vi "RunFullWormRails.vi"() -> ()   [LabVIEW 2019]
uses:
  Parameters.ctl
  FullWormRails/FullWormRailsInputCluster.ctl
  FullWormRails.lvclass
  D:/Github_repos/ProjectAPI/LabviewVIs/StimulusObject.lvclass
panel:
  in  "FullWormRailsInputCluster":T1={"Constant Intensity (uW/mm^2, negative is blue)"=0.0, "dot radius (mm)"=0.3, "Intensities (uW/mm^2, negative is blue)"=[], "Durations (s)"=[], "Inter trigger interval (s)"=10.0}
  out "error IO":errorcluster
  in  "SSH password 2":string
  in  "SSH user name 2":string
  in  "Start":bool
  in  "Wait Before Recording (s)":u32
  in  "SSH password":string
  in  "username@della.princeton.edu":string
  in  "Last Experiment of the Day":bool
  in  "Tags":string
  out "Parameters":T2 {"FW_WormLengthSD" format="%#.6e"}
  # "Faux Worm Drawing"
  # "Tracking"
  # "Temporal Calibration"
  # "Stimulus Generation"
  # "Median Filtering"
  # "Experimental Settings"
  # "Camera and Projector Settings"
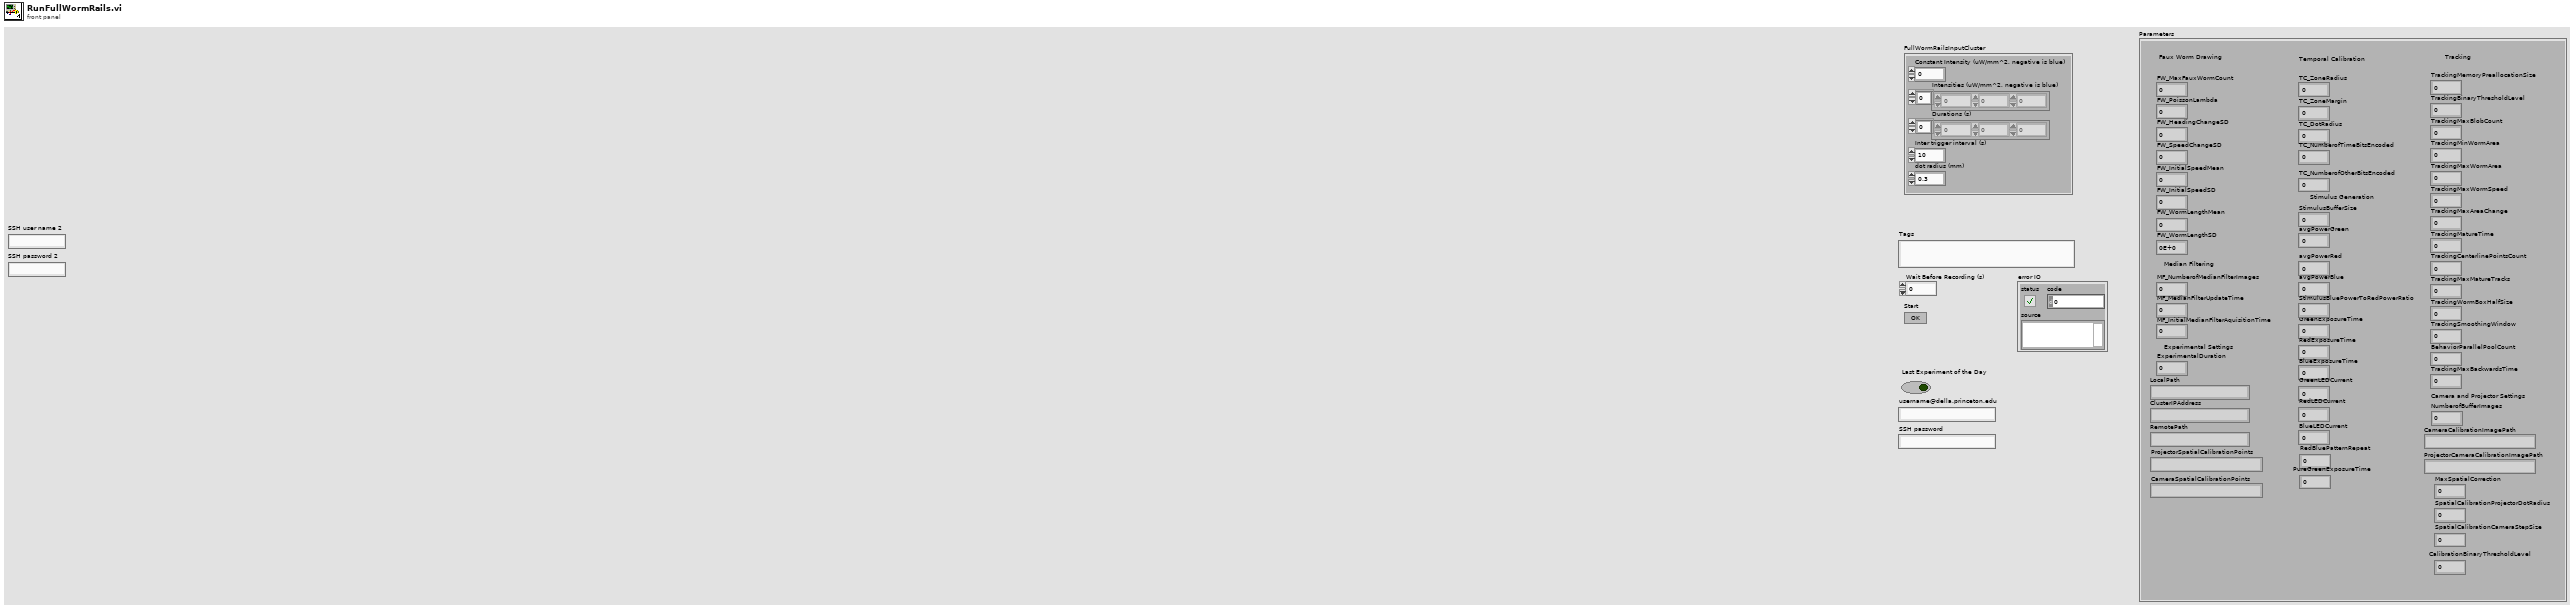
[diagram p1: front panel]
types:
  T1 = typedef "FullWormRails.lvclass/FullWormRailsInputCluster.ctl" = cluster{"Constant Intensity (uW/mm^2, negative is blue)":sgl, "dot radius (mm)":sgl, "Intensities (uW/mm^2, negative is blue)":sgl[], "Durations (s)":sgl[], "Inter trigger interval (s)":dbl}
  T2 = typedef "Parameters.ctl" = cluster{"FW_MaxFauxWormCount":i32, "FW_PoissonLambda":dbl, "FW_HeadingChangeSD":dbl, "FW_SpeedChangeSD":dbl, "FW_InitialSpeedMean":dbl, "FW_InitialSpeedSD":dbl, "FW_WormLengthMean":dbl, "FW_WormLengthSD":dbl, "MF_NumberofMedianFilterImages":i32, "MF_MedianFilterUpdateTime":i32, "MF_InitialMedianFilterAquisitionTime":dbl, "ExperimentalDuration":i32, "TC_ZoneRadius":i32, "TC_ZoneMargin":i32, "TC_DotRadius":dbl, "TC_NumberofTimeBitsEncoded":i32, "TC_NumberofOtherBitsEncoded":i32, "NumberofBufferImages":sgl, "CameraCalibrationImagePath":string, "ProjectorCameraCalibrationImagePath":string, "StimulusBufferSize":i32, "TrackingMemoryPreallocationSize":i32, "TrackingBinaryThresholdLevel":sgl, "TrackingMaxBlobCount":i32, "TrackingMinWormArea":dbl, "TrackingMaxWormArea":dbl, "TrackingMaxWormSpeed":dbl, "TrackingMaxAreaChange":dbl, "TrackingMatureTime":i32, "TrackingCenterlinePointsCount":i32, "TrackingMaxMatureTracks":i32, "TrackingWormBoxHalfSize":i32, "TrackingSmoothingWindow":i32, "BehaviorParallelPoolCount":i32, "LocalPath":string, "GreenExposureTime":i32, "RedExposureTime":i32, "BlueExposureTime":i32, "ClusterIPAddress":string, "RemotePath":string, "GreenLEDCurrent":u8, "RedLEDCurrent":u8, "BlueLEDCurrent":u8, "avgPowerGreen":sgl, "avgPowerRed":sgl, "avgPowerBlue":sgl, "StimulusBluePowerToRedPowerRatio":sgl, "TrackingMaxBackwardsTime":i32, "MaxSpatialCorrection":dbl, "ProjectorSpatialCalibrationPoints":string, "SpatialCalibrationProjectorDotRadius":i32, "SpatialCalibrationCameraStepSize":dbl, "CameraSpatialCalibrationPoints":string, "CalibrationBinaryThresholdLevel":dbl, "RedBluePatternRepeat":i32, "PureGreenExposureTime":i32}
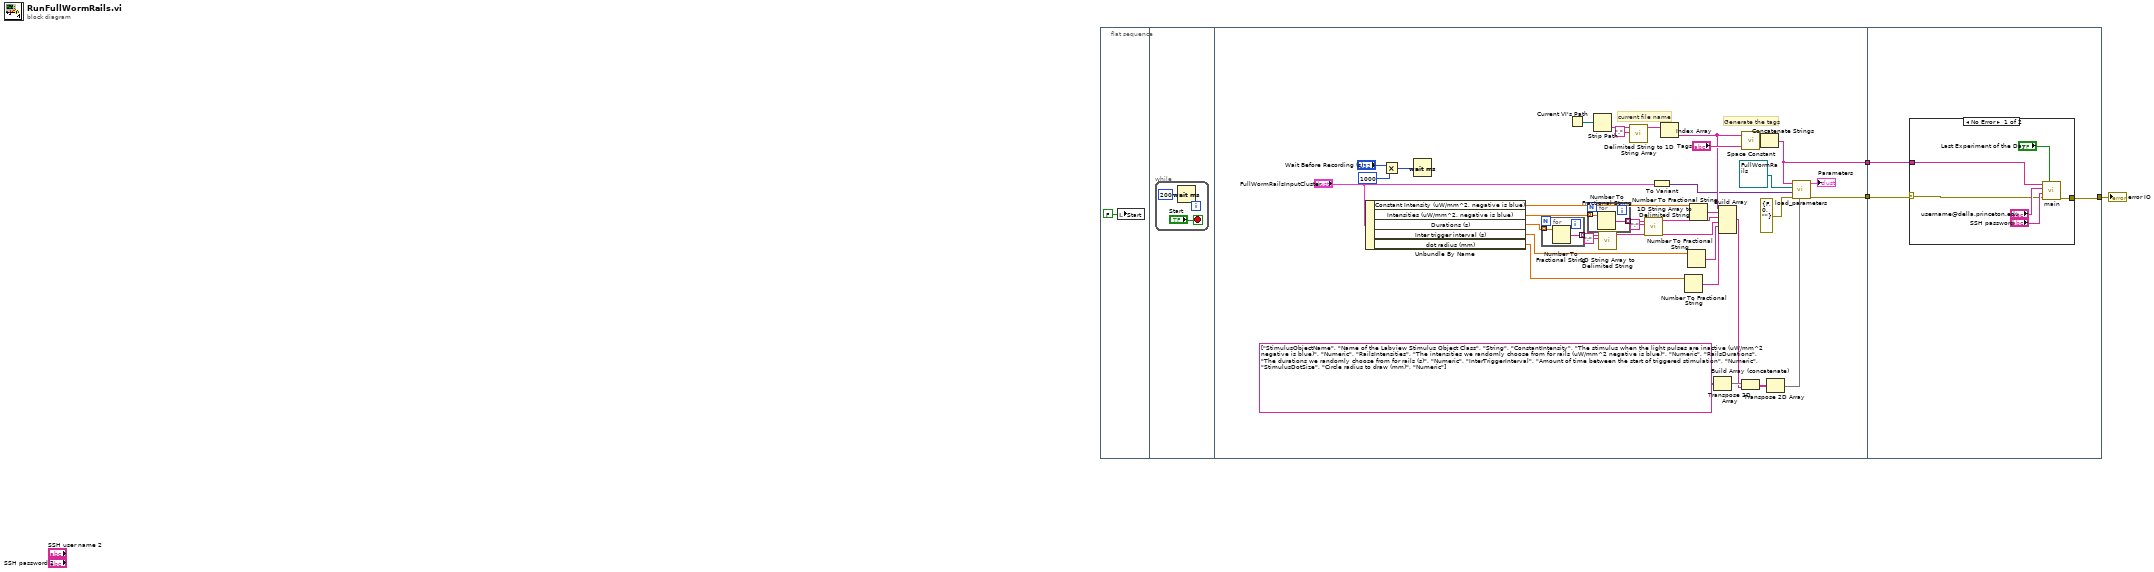
[diagram p0: block diagram]
diagram:
  n1 = flat-sequence {
    tunnel: [w42] -> w3
    tunnel: [w32] -> w2
    tunnel: w2 -> [w48]
    tunnel: w3 -> [w49]
    tunnel: [w47] -> w1
    frame #0 {
      n2 = local write "Start"(FALSE ("Start")) -> ()
    }
    frame #1 {
      n3 = while {
        stop <- "Start" stop-if-true
        n4 = Wait (ms)(milliseconds to wait=u32 200) -> ()  [unwired: 1 out]
      }
    }
    frame #2 {
      # "current file name"
      # "Generate the tags"
      n5 = Unbundle By Name("FullWormRailsInputCluster") -> ("Constant Intensity (uW/mm^2, negative is blue)"=w20:sgl, "Intensities (uW/mm^2, negative is blue)"=w19:sgl[], "Durations (s)"=w13:sgl[], "Inter trigger interval (s)"=w10:dbl, "dot radius (mm)"=w11:sgl)
      n6 = Multiply(x="Wait Before Recording (s)", y=u32 1000) -> (x*y=w29:u32)
      n7 = Wait (ms)(milliseconds to wait=w29) -> ()  [unwired: 1 out]
      n8 = for {
        tunnel: w13 -> [w44] mode=indexing
        tunnel: [w43] -> w15 mode=indexing
        n9 = Number To Fractional String(number=w44) -> (F-format string=w43:string)  [unwired: 3 in]
      }
      n10 = Current VI's Path() -> (path=w27:path)
      n11 = for {
        tunnel: w19 -> [w46] mode=indexing
        tunnel: [w45] -> w18 mode=indexing
        n12 = Number To Fractional String(number=w46) -> (F-format string=w45:string)  [unwired: 3 in]
      }
      n13 = Strip Path(path=w27) -> (name=w26:string)  [unwired: 1 out]
      n14 = call <vilib>:"1D String Array to Delimited String.vi"("delimiter"=";", "string array"=w15) -> ("delimited string"=w12:string)  [unwired: 9 in]
      n15 = call <vilib>:"Delimited String to 1D String Array.vi"("delimiter"=".", "delimited string"=w26) -> ("string array"=w24:string[])  [unwired: 9 in]
      n16 = call <vilib>:"1D String Array to Delimited String.vi"("delimiter"=";", "string array"=w18) -> ("delimited string"=w16:string)  [unwired: 9 in]
      n17 = To Variant(anything="FullWormRailsInputCluster") -> (Variant=w22:variant)
      n18 = Index Array(array=w24) -> (element=w23:string)  [unwired: 1 in]
      n19 = Number To Fractional String(number=w11) -> (F-format string=w8:string)  [unwired: 3 in]
      n20 = Number To Fractional String(number=w10) -> (F-format string=w9:string)  [unwired: 3 in]
      n21 = Number To Fractional String(number=w20) -> (F-format string=w40:string)  [unwired: 3 in]
      n22 = Transpose 2D Array(2D array=string[][] [["StimulusObjectName", "Name of the Labview Stimulus Object Class", "String"], ["ConstantIntensity", "The stimulus when the light pulses are inactive (uW/mm^2 negative is blue)", "Numeric"], ["RailsIntensities", "The intensities we randomly choose from for rails (uW/mm^2 negative is blue)", "Numeric"], ["RailsDurations", "The durations we randomly choose from for rails (s)", "Numeric"], ["InterTriggerInterval", "Amount of time between the start of triggered stimulation", "Numeric"], ["StimulusDotSize", "Circle radius to draw (mm)", "Numeric"]]) -> (transposed array=w38:string[][])
      n23 = Build Array(w23, w40, w16, w12, w9, w8) -> (w37:string[])
      n24 = Build Array (concatenate)(w38, w37) -> (w36:string[][])
      n25 = call <vilib>:"Space Constant.vi"() -> ("String"=w34:string)
      n26 = Concatenate Strings(w23, w34, "Tags") -> (w32:string)
      n27 = Transpose 2D Array(2D array=w36) -> (transposed array=w33:string[][])
      n28 = call "load_parameters.vi"("additional loaded parameters to write"=w33, "error in (no error)"=errorcluster {"status"=FALSE, "code"=0, "source"=""}, "StimulusObject Parameters"=w22, "StimulusObjectClassInput"=refnum<class "FullWormRails.lvclass"> refnum ("FullWormRails.lvclass"), "Tags"=w32) -> ("error out"=w42:errorcluster, "Parameters"=→"Parameters":T2)  [unwired: 4 in, 1 out]
    }
    frame #3 {
      n29 = case shown="No Error" w49 {
        selector: w49 -> [w52 w56]
        tunnel: [w51 w56] -> w47
        tunnel: w48 -> [w50 _]
        frame No Error {
          n30 = call "main.vi"("Last Experiment of the Day"="Last Experiment of the Day", "error in"=w52, "SSH password"="SSH password", "SSH user name"="username@della.princeton.edu", "Tags"=w50) -> ("error out"=w51:errorcluster)  [unwired: 6 in]
        }
        frame Error {
        }
      }
    }
  }
  "error IO" <- w1
